vi "GUI.vi"() -> ()   [LabVIEW 2020]
uses:
  <vilib>/Utility/miscctls.llb/LVForegroundBackgroundColorsTypeDef.ctl
  <vilib>/Utility/config.llb/Write Key (String).vi
  <vilib>/Utility/config.llb/Write Key (Boolean).vi
  <vilib>/Utility/config.llb/Write Key (Double).vi
  <vilib>/Utility/config.llb/Write Key (U32).vi
  <vilib>/Utility/config.llb/Read Key (String).vi
  <vilib>/Utility/config.llb/Read Key (Boolean).vi
  <vilib>/Utility/config.llb/Read Key (U32).vi
  <vilib>/Utility/config.llb/Read Key (Double).vi
  <vilib>/Utility/config.llb/NI_LVConfig.lvlib
panel:
  in  "load profiles":bool
  in  "Profile name":string
  in  "Saved profiles":string(combo)
  in  "Save Button":bool
  in  "# channels":dbl=4.0 min=3.0 max=4.0 format="%#_1g"
  in  "To be ignored":dbl=3.0 min=1.0 max=4.0 step=1.0
  in  "RED":dbl=4.0 min=1.0 max=4.0 step=1.0
  in  "GREEN":dbl=1.0 min=1.0 max=4.0 step=1.0
  in  "BLUE":dbl=2.0 min=1.0 max=4.0 step=1.0
  in  "block size":dbl=101.0
  in  "Scroll to last":bool
  in  "Remove Button":bool
  out "Final Scroll Position":i32
  in  "Initial Scroll Position":u32
  out "messages":string
  in  "Red Ch.":bool=TRUE
  in  "Blue Ch.":bool
  in  "Green Ch.":bool=TRUE
  in  "Detailed output":bool
  in  "Python version":string="3.9"
  out "Warning":bool
  out "Error":bool
  out "Warning and error window":string
  out "green static indicator":bool
  out "blue static indicator":bool
  out "red static indicator":bool
  out "Saving":bool
  in  "Overlay Transparency":dbl=0.5 min=0.0 max=1.0 format="%#_3g"
  in  "Activate":bool
  in  "Green":bool
  in  "Blue":bool
  in  "Red":bool
  in  "Green":dbl min=0.0 step=0.001 format="%#_3g"
  in  "Blue":dbl=0.03 min=0.0 step=0.001 format="%#_3g"
  in  "Red":dbl min=0.0 step=0.001 format="%#.3g"
  in  "Green":dbl min=0.0 step=0.001 format="%#_3g"
  in  "Blue":dbl=0.03 min=0.0 step=0.001 format="%#_3g"
  in  "Red":dbl min=0.0 step=0.001 format="%#.3g"
  in  "Green":dbl=1.5 format="%#_2g"
  in  "Blue":dbl=1.5 format="%_2g"
  in  "Red":dbl=1.5 format="%.1g"
  in  "Activate":bool
  in  "Green":dbl=4.0 min=1.0 step=1.0 format="%#_1f"
  in  "Blue":dbl=4.0 min=1.0 step=1.0 format="%_1f"
  in  "Red":dbl=2.0 min=1.0 step=1.0
  in  "Green":bool=TRUE
  in  "Blue":bool=TRUE
  in  "Red":bool=TRUE
  in  "Border thickness (single channel) 2":dbl=1.0 min=1.0 step=1.0 format="%#_3g"
  in  "Activate":bool
  in  "Blue Ch":u32(colorbox)=16711680
  in  "Green Ch":u32(colorbox)=65280
  in  "Red Ch":u32(colorbox)=255
  in  "Red Ch":u32(colorbox)=16776960
  in  "Green Ch":u32(colorbox)=12357519
  in  "Blue Ch":u32(colorbox)=16777215
  in  "Red":dbl=20.0 min=1.0 max=255.0
  in  "Blue":dbl=20.0 min=1.0 max=255.0 format="%_1f"
  in  "Green":dbl=20.0 min=1.0 max=255.0 format="%#_1f"
  in  "Red":dbl=2.0
  in  "Blue":dbl format="%_1f"
  in  "Green":dbl=1.0 format="%#_1f"
  in  "Red":dbl=30000.0 min=2.0 step=1.0
  in  "Blue":dbl=30000.0 min=2.0 step=1.0 format="%_1f"
  in  "Green":dbl=30000.0 min=2.0 step=1.0 format="%#_1f"
  in  "Red":dbl=40.0 min=1.0 step=1.0
  in  "Blue":dbl=40.0 min=1.0 step=1.0 format="%_1f"
  in  "Green":dbl=40.0 min=1.0 step=1.0 format="%#_1f"
  in  "Filling contours by solid color":bool=TRUE
  in  "Border thickness (overlay)":dbl=1.0 format="%#_3g"
  in  "Border thickness (single channel)":dbl=1.0 format="%#_3g"
  in  "General border color":u32(colorbox)=16777215
  in  "Number of bins":dbl=10.0 min=1.0 step=1.0 format="%#_3g"
  out "Processing":bool
  in  "Run":bool
  in  "Green":dbl=2.0 min=1.0 max=3.0 step=1.0 format="%#_1f"
  in  "Blue":dbl=1.0 min=1.0 max=3.0 step=1.0 format="%#_1g"
  in  "Red":dbl=3.0 min=1.0 max=3.0 step=1.0
  in  "Activate Histogram":bool
  in  "Input folder":string="images/"
  in  "Zero Pixel Reporter":bool
  in  "Contour Detail Reporter":bool
  in  "Transparent Corrector":bool=TRUE
  in  "Save":bool
  # "Path information"
  # "Morphological Filter (ellipse and circular)"
  # "Thresholds"
  # "Color Recipe"
  # "Advance Tools"
  # "Global"
  # "Channel to proccess"
  # "Elliptical Ratio Filter"
  # "Biggest contour generator"
  # "Adaptive"
  # "Circular Ratio Filter"
  # "Up to"
  # "biggest"
  # "Morphological Filter (Ratio)"
  # "Order of plot in histogram"
  # "Visual Effects"
  # "Border colors in full map"
  # "Border colors in transparent map"
  # "Selection Filter"
  # "Block Size"
  # "Size Filter"
  # "Process Order"
  # "Messages:"
  # "Minimum size limit"
  # "Maximum size limit"
  # "Designed by Shahab Bahreini"
  # "Warnings:"
  # "ver. 2.0.0"
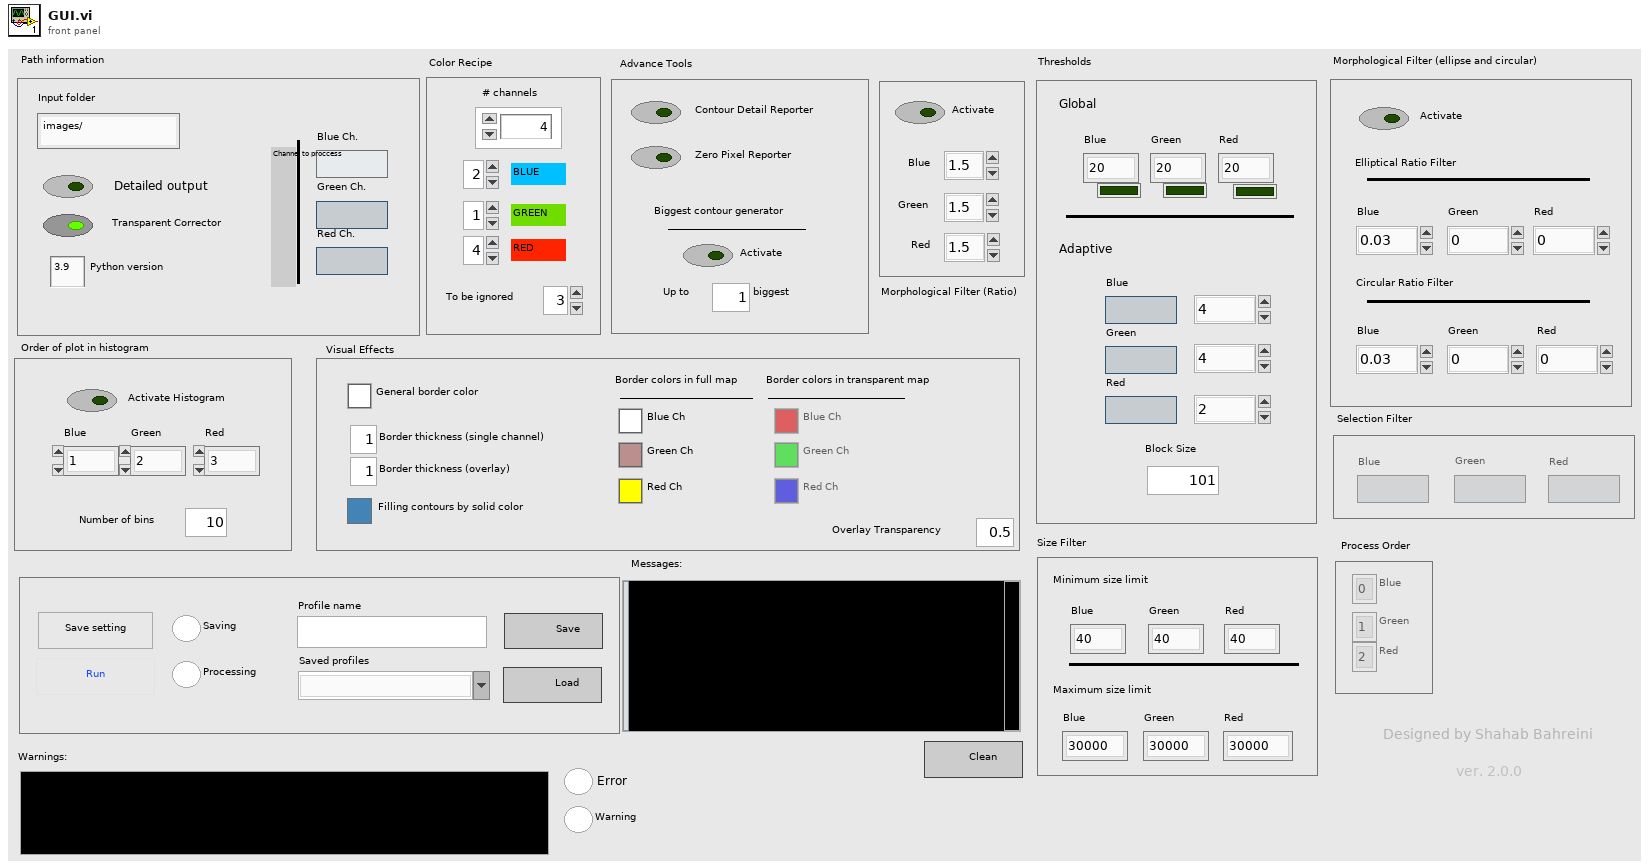
[diagram p1: front panel]
types:
  T1 = enum8{"Enabled", "Disabled", "Disabled and Grayed Out"}
  T2 = typedef "LVForegroundBackgroundColorsTypeDef.ctl" = cluster{"Foreground Color":u32, "Background Color":u32}
  T3 = typedef "NI_LVConfig.lvlib/Config Data RefNum.ctl" = refnum<k1>
  T4 = enum16{"open", "replace", "create", "open or create", "replace or create", "replace or create with confirmation"}
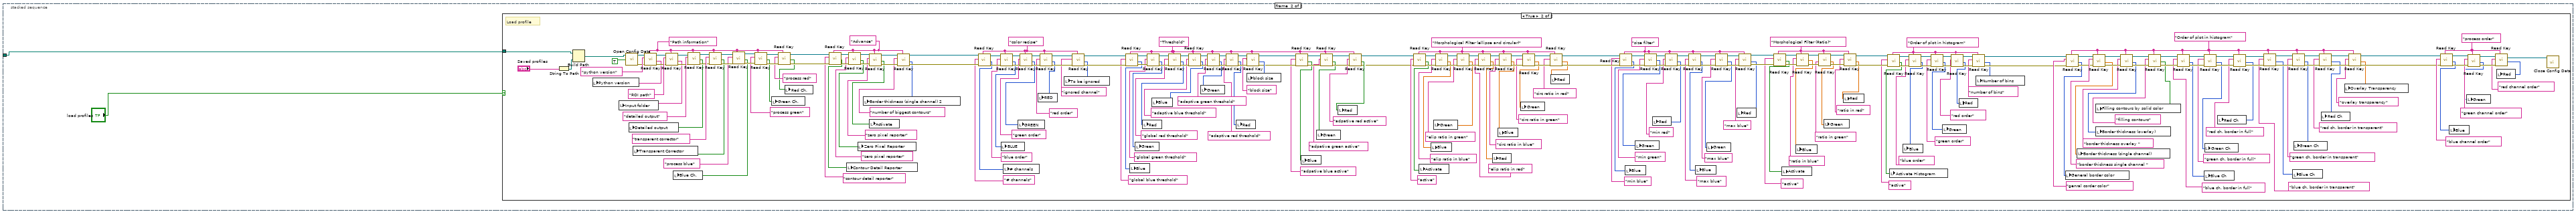
[diagram p3: hidden frame]
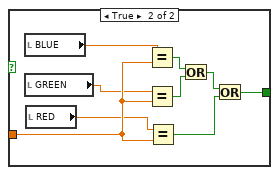
[diagram p5: hidden frame]
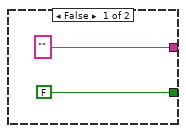
[diagram p6: hidden frame]
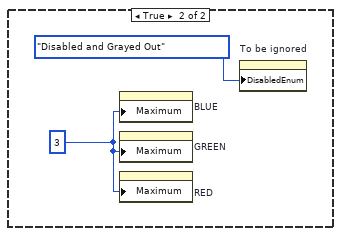
[diagram p7: hidden frame]
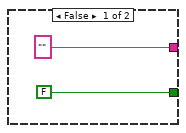
[diagram p9: hidden frame]
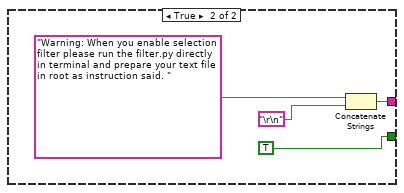
[diagram p10: hidden frame]
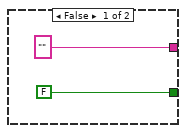
[diagram p11: hidden frame]
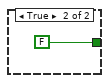
[diagram p12: hidden frame]
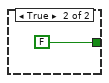
[diagram p13: hidden frame]
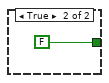
[diagram p14: hidden frame]
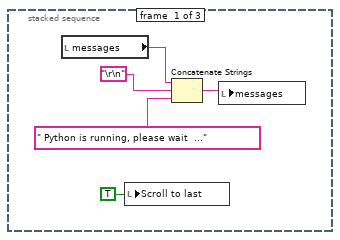
[diagram p16: hidden frame]
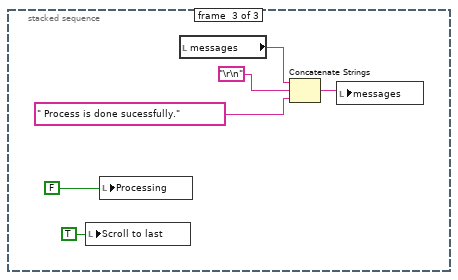
[diagram p17: hidden frame]
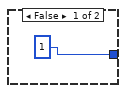
[diagram p19: hidden frame]
diagram:
  # "Finds all .ini profiles"
  # "Recepie error checker"
  # "Selection filter checker"
  # "Size limit checker"
  # "Order of plot checker"
  n1 = local read "Warning and error window"() -> (→"Warning and error window":string)
  n2 = property on="Warning and error window" class="Str"("Text.FontBold"=FALSE ("Text.Font:Bold")) -> ()  [unwired: 2 in, 2 out]
  n3 = property on="Warning and error window" class="Str"("Text.Colors"=T2 {"Foreground Color"=0, "Background Color"=16777222}) -> ()  [unwired: 2 in, 2 out]
  n4 = Equal?(x="# channels", y=3.0) -> (x = y?=w25:bool)
  n5 = case shown="False" w25 {
    frame False {
      w77 = 4
      n6 = property on="BLUE" class="DigNum (strict)"("Maximum"=w77) -> ()  [unwired: 2 in, 2 out]
      n7 = property on="GREEN" class="DigNum (strict)"("Maximum"=w77) -> ()  [unwired: 2 in, 2 out]
      n8 = property on="RED" class="DigNum (strict)"("Maximum"=w77) -> ()  [unwired: 2 in, 2 out]
      n9 = property on="To be ignored" class="DigNum (strict)"("DisabledEnum"=T1."Enabled" ("Disabled")) -> ()  [unwired: 2 in, 2 out]
    }
    frame True {
      w79 = 3
      n10 = property on="BLUE" class="DigNum (strict)"("Maximum"=w79) -> ()  [unwired: 2 in, 2 out]
      n11 = property on="GREEN" class="DigNum (strict)"("Maximum"=w79) -> ()  [unwired: 2 in, 2 out]
      n12 = property on="RED" class="DigNum (strict)"("Maximum"=w79) -> ()  [unwired: 2 in, 2 out]
      n13 = property on="To be ignored" class="DigNum (strict)"("DisabledEnum"=T1."Disabled and Grayed Out" ("Disabled")) -> ()  [unwired: 2 in, 2 out]
    }
  }
  n14 = Current VI's Path() -> (path=w4:path)
  n15 = Strip Path(path=w4) -> (stripped path=w3:path)  [unwired: 1 out]
  n16 = local read "Green"() -> (w71:bool)
  n17 = local read "Blue"() -> (w70:bool)
  n18 = local read "Red"() -> (w72:bool)
  n19 = Build Path(base path=w3, name or relative path=path "profiles") -> (appended path=w1:path)
  n20 = case shown="False" w70 {
    tunnel: [TRUE ("Boolean") FALSE ("Boolean")] -> w68
    frame False {
    }
    frame True {
    }
  }
  "blue static indicator" <- w68
  n21 = case shown="False" w72 {
    tunnel: [TRUE ("Boolean") FALSE ("Boolean")] -> w73
    frame False {
    }
    frame True {
    }
  }
  "red static indicator" <- w73
  n22 = List Folder(path=w1) -> (filenames=w5:string[])  [unwired: 3 in, 3 out]
  n23 = case shown="False" w71 {
    tunnel: [TRUE ("Boolean") FALSE ("Boolean")] -> w69
    frame False {
    }
    frame True {
    }
  }
  "green static indicator" <- w69
  n24 = property on="Saved profiles" class="CmbBox"("Strings[]"=w5) -> ()  [unwired: 2 in, 2 out]
  n25 = local read "To be ignored"() -> (w11:dbl)
  n26 = property on="To be ignored" class="DigNum (strict)"() -> ("DisabledEnum"=w14:T1)  [unwired: 2 in, 2 out]
  n27 = stacked-sequence {
    tunnel: w1 -> [w87 w353]
    frame #0 {
      n28 = case shown="True" "Save Button" {
        tunnel: w87 -> [_ w335]
        frame False {
        }
        frame True {
          w113 = "process order" ("section")
          w142 = "Order of plot in histogram" ("section")
          w183 = "Order of plot in histogram" ("section")
          w184 = "Morphological Filter (Ratio)" ("section")
          w215 = "size filter" ("section")
          w252 = "Morphological Filter (ellipse and circular)" ("section")
          w93 = "Threshold" ("section")
          w279 = "color recipe" ("section")
          w300 = "Advance" ("section")
          w318 = "Path information" ("section")
          # "Save profile"
          n29 = Concatenate Strings("Profile name", ".ini" ("string")) -> (w338:string)
          n30 = String To Path(string=w338) -> (path=w337:path)
          n31 = Build Path(base path=w335, name or relative path=w337) -> (appended path=w340:path)
          n32 = local read "Python version"() -> (w317:string)
          n33 = local read "Input folder"() -> (w345:string)
          n34 = call <vilib>:"Open Config Data.vi"("create file if necessary (T)"=TRUE, "configuration file path"=w340) -> ("error out"=w332:errorcluster, "refnum"=w349:T3)  [unwired: 7 in, 1 out]
          n35 = local read "Detailed output"() -> (w344:bool)
          n36 = local read "Transparent Corrector"() -> (w341:bool)
          n37 = call-poly <vilib>:"Write Key.vi"("section"=w318, "error in (no error)"=w332, "value"=w317, "key"="python version", "refnum"=w349) -> ("error out"=w331:errorcluster, "refnum out"=w352:T3)  [unwired: 4 in, 1 out]
          n38 = local read "Blue Ch."() -> (w327:bool)
          n39 = call-poly <vilib>:"Write Key.vi"("section"=w318, "error in (no error)"=w331, "value"=w345, "key"="ROI path", "refnum"=w352) -> ("error out"=w330:errorcluster, "refnum out"=w351:T3)  [unwired: 4 in, 1 out]
          n40 = call-poly <vilib>:"Write Key.vi"("section"=w318, "error in (no error)"=w330, "value"=w344, "key"="detailed output", "refnum"=w351) -> ("error out"=w329:errorcluster, "refnum out"=w350:T3)  [unwired: 4 in, 1 out]
          n41 = call-poly <vilib>:"Write Key.vi"("section"=w318, "error in (no error)"=w329, "value"=w341, "key"="transparent corrector", "refnum"=w350) -> ("error out"=w334:errorcluster, "refnum out"=w333:T3)  [unwired: 4 in, 1 out]
          n42 = call-poly <vilib>:"Write Key.vi"("section"=w318, "error in (no error)"=w334, "value"=w327, "key"="process blue", "refnum"=w333) -> ("error out"=w324:errorcluster, "refnum out"=w326:T3)  [unwired: 4 in, 1 out]
          n43 = local read "Green Ch."() -> (w319:bool)
          n44 = call-poly <vilib>:"Write Key.vi"("section"=w318, "error in (no error)"=w324, "value"=w319, "key"="process green", "refnum"=w326) -> ("error out"=w323:errorcluster, "refnum out"=w325:T3)  [unwired: 4 in, 1 out]
          n45 = local read "Red Ch."() -> (w321:bool)
          n46 = call-poly <vilib>:"Write Key.vi"("section"=w318, "error in (no error)"=w323, "value"=w321, "key"="process red", "refnum"=w325) -> ("error out"=w315:errorcluster, "refnum out"=w316:T3)  [unwired: 4 in, 1 out]
          n47 = local read "Contour Detail Reporter"() -> (w314:bool)
          n48 = call-poly <vilib>:"Write Key.vi"("section"=w300, "error in (no error)"=w315, "value"=w314, "key"="contour detail reporter", "refnum"=w316) -> ("error out"=w312:errorcluster, "refnum out"=w311:T3)  [unwired: 4 in, 1 out]
          n49 = local read "Zero Pixel Reporter"() -> (w309:bool)
          n50 = call-poly <vilib>:"Write Key.vi"("section"=w300, "error in (no error)"=w312, "value"=w309, "key"="zero pixel reporter", "refnum"=w311) -> ("error out"=w308:errorcluster, "refnum out"=w307:T3)  [unwired: 4 in, 1 out]
          n51 = local read "Activate"() -> (w306:bool)
          n52 = local read "Border thickness (single channel) 2"() -> (w302:dbl)
          n53 = call-poly <vilib>:"Write Key.vi"("section"=w300, "error in (no error)"=w308, "value"=w306, "key"="zero pixel reporter", "refnum"=w307) -> ("error out"=w304:errorcluster, "refnum out"=w303:T3)  [unwired: 4 in, 1 out]
          n54 = call-poly <vilib>:"Write Key.vi"("section"=w300, "error in (no error)"=w304, "value"=w302, "key"="number of biggest contours", "refnum"=w303) -> ("error out"=w295:errorcluster, "refnum out"=w296:T3)  [unwired: 4 in, 1 out]
          n55 = local read "BLUE"() -> (w289:dbl)
          n56 = local read "# channels"() -> (w291:dbl)
          n57 = call-poly <vilib>:"Write Key.vi"("section"=w279, "error in (no error)"=w295, "value"=w291, "key"="# channels", "refnum"=w296) -> ("error out"=w294:errorcluster, "refnum out"=w299:T3)  [unwired: 4 in, 1 out]
          n58 = call-poly <vilib>:"Write Key.vi"("section"=w279, "error in (no error)"=w294, "value"=w289, "key"="blue order", "refnum"=w299) -> ("error out"=w293:errorcluster, "refnum out"=w298:T3)  [unwired: 4 in, 1 out]
          n59 = local read "GREEN"() -> (w286:dbl)
          n60 = call-poly <vilib>:"Write Key.vi"("section"=w279, "error in (no error)"=w293, "value"=w286, "key"="green order", "refnum"=w298) -> ("error out"=w292:errorcluster, "refnum out"=w297:T3)  [unwired: 4 in, 1 out]
          n61 = local read "RED"() -> (w285:dbl)
          n62 = call-poly <vilib>:"Write Key.vi"("section"=w279, "error in (no error)"=w292, "value"=w285, "key"="red order", "refnum"=w297) -> ("error out"=w283:errorcluster, "refnum out"=w282:T3)  [unwired: 4 in, 1 out]
          n63 = local read "To be ignored"() -> (w281:dbl)
          n64 = call-poly <vilib>:"Write Key.vi"("section"=w279, "error in (no error)"=w283, "value"=w281, "key"="ignored channel", "refnum"=w282) -> ("error out"=w267:errorcluster, "refnum out"=w268:T3)  [unwired: 4 in, 1 out]
          n65 = local read "Blue"() -> (w265:dbl)
          n66 = call-poly <vilib>:"Write Key.vi"("section"=w93, "error in (no error)"=w267, "value"=w265, "key"="global blue threshold", "refnum"=w268) -> ("error out"=w273:errorcluster, "refnum out"=w275:T3)  [unwired: 4 in, 1 out]
          n67 = local read "Green"() -> (w263:dbl)
          n68 = local read "Red"() -> (w261:dbl)
          n69 = local read "Blue"() -> (w260:dbl)
          n70 = call-poly <vilib>:"Write Key.vi"("section"=w93, "error in (no error)"=w273, "value"=w263, "key"="global green threshold", "refnum"=w275) -> ("error out"=w272:errorcluster, "refnum out"=w276:T3)  [unwired: 4 in, 1 out]
          n71 = call-poly <vilib>:"Write Key.vi"("section"=w93, "error in (no error)"=w272, "value"=w261, "key"="global red threshold", "refnum"=w276) -> ("error out"=w271:errorcluster, "refnum out"=w277:T3)  [unwired: 4 in, 1 out]
          n72 = call-poly <vilib>:"Write Key.vi"("section"=w93, "error in (no error)"=w271, "value"=w260, "key"="adaptive blue threshold", "refnum"=w277) -> ("error out"=w270:errorcluster, "refnum out"=w278:T3)  [unwired: 4 in, 1 out]
          n73 = local read "Red"() -> (w256:dbl)
          n74 = local read "block size"() -> (w254:dbl)
          n75 = local read "Green"() -> (w258:dbl)
          n76 = call-poly <vilib>:"Write Key.vi"("section"=w93, "error in (no error)"=w270, "value"=w258, "key"="adaptive green threshold", "refnum"=w278) -> ("error out"=w92:errorcluster, "refnum out"=w96:T3)  [unwired: 4 in, 1 out]
          n77 = call-poly <vilib>:"Write Key.vi"("section"=w93, "error in (no error)"=w92, "value"=w256, "key"="adaptive red threshold", "refnum"=w96) -> ("error out"=w269:errorcluster, "refnum out"=w274:T3)  [unwired: 4 in, 1 out]
          n78 = call-poly <vilib>:"Write Key.vi"("section"=w93, "error in (no error)"=w269, "value"=w254, "key"="block size", "refnum"=w274) -> ()  [unwired: 4 in, 3 out]
          n79 = local read "Blue"() -> (w91:bool)
          n80 = call-poly <vilib>:"Write Key.vi"("section"=w93, "error in (no error)"=w92, "value"=w91, "key"="adpative blue active", "refnum"=w96) -> ("error out"=w101:errorcluster, "refnum out"=w103:T3)  [unwired: 4 in, 1 out]
          n81 = local read "Green"() -> (w90:bool)
          n82 = call-poly <vilib>:"Write Key.vi"("section"=w93, "error in (no error)"=w101, "value"=w90, "key"="adpative green active", "refnum"=w103) -> ("error out"=w100:errorcluster, "refnum out"=w102:T3)  [unwired: 4 in, 1 out]
          n83 = local read "Red"() -> (w89:bool)
          n84 = call-poly <vilib>:"Write Key.vi"("section"=w93, "error in (no error)"=w100, "value"=w89, "key"="adpative red active", "refnum"=w102) -> ("error out"=w94:errorcluster, "refnum out"=w95:T3)  [unwired: 4 in, 1 out]
          n85 = local read "Activate"() -> (w238:bool)
          n86 = call-poly <vilib>:"Write Key.vi"("section"=w252, "error in (no error)"=w94, "value"=w238, "key"="active", "refnum"=w95) -> ("error out"=w246:errorcluster, "refnum out"=w243:T3)  [unwired: 4 in, 1 out]
          n87 = local read "Blue"() -> (w236:dbl)
          n88 = local read "Green"() -> (w235:dbl)
          n89 = call-poly <vilib>:"Write Key.vi"("section"=w252, "error in (no error)"=w246, "value"=w236, "key"="elip ratio in blue", "refnum"=w243) -> ("error out"=w247:errorcluster, "refnum out"=w242:T3)  [unwired: 4 in, 1 out]
          n90 = call-poly <vilib>:"Write Key.vi"("section"=w252, "error in (no error)"=w247, "value"=w235, "key"="elip ratio in green", "refnum"=w242) -> ("error out"=w248:errorcluster, "refnum out"=w241:T3)  [unwired: 4 in, 1 out]
          n91 = local read "Red"() -> (w233:dbl)
          n92 = call-poly <vilib>:"Write Key.vi"("section"=w252, "error in (no error)"=w248, "value"=w233, "key"="elip ratio in red", "refnum"=w241) -> ("error out"=w249:errorcluster, "refnum out"=w240:T3)  [unwired: 4 in, 1 out]
          n93 = local read "Blue"() -> (w230:dbl)
          n94 = call-poly <vilib>:"Write Key.vi"("section"=w252, "error in (no error)"=w249, "value"=w230, "key"="circ ratio in blue", "refnum"=w240) -> ("error out"=w250:errorcluster, "refnum out"=w245:T3)  [unwired: 4 in, 1 out]
          n95 = local read "Green"() -> (w229:dbl)
          n96 = call-poly <vilib>:"Write Key.vi"("section"=w252, "error in (no error)"=w250, "value"=w229, "key"="circ ratio in green", "refnum"=w245) -> ("error out"=w251:errorcluster, "refnum out"=w244:T3)  [unwired: 4 in, 1 out]
          n97 = local read "Red"() -> (w226:dbl)
          n98 = call-poly <vilib>:"Write Key.vi"("section"=w252, "error in (no error)"=w251, "value"=w226, "key"="circ ratio in red", "refnum"=w244) -> ("error out"=w213:errorcluster, "refnum out"=w214:T3)  [unwired: 4 in, 1 out]
          n99 = local read "Blue"() -> (w211:dbl)
          n100 = call-poly <vilib>:"Write Key.vi"("section"=w215, "error in (no error)"=w213, "value"=w211, "key"="min blue", "refnum"=w214) -> ("error out"=w220:errorcluster, "refnum out"=w223:T3)  [unwired: 4 in, 1 out]
          n101 = local read "Green"() -> (w209:dbl)
          n102 = call-poly <vilib>:"Write Key.vi"("section"=w215, "error in (no error)"=w220, "value"=w209, "key"="min green", "refnum"=w223) -> ("error out"=w219:errorcluster, "refnum out"=w224:T3)  [unwired: 4 in, 1 out]
          n103 = local read "Red"() -> (w208:dbl)
          n104 = call-poly <vilib>:"Write Key.vi"("section"=w215, "error in (no error)"=w219, "value"=w208, "key"="min red", "refnum"=w224) -> ("error out"=w218:errorcluster, "refnum out"=w225:T3)  [unwired: 4 in, 1 out]
          n105 = local read "Blue"() -> (w205:dbl)
          n106 = call-poly <vilib>:"Write Key.vi"("section"=w215, "error in (no error)"=w218, "value"=w205, "key"="max blue", "refnum"=w225) -> ("error out"=w217:errorcluster, "refnum out"=w221:T3)  [unwired: 4 in, 1 out]
          n107 = local read "Green"() -> (w203:dbl)
          n108 = call-poly <vilib>:"Write Key.vi"("section"=w215, "error in (no error)"=w217, "value"=w203, "key"="max blue", "refnum"=w221) -> ("error out"=w216:errorcluster, "refnum out"=w222:T3)  [unwired: 4 in, 1 out]
          n109 = local read "Red"() -> (w201:dbl)
          n110 = call-poly <vilib>:"Write Key.vi"("section"=w215, "error in (no error)"=w216, "value"=w201, "key"="max blue", "refnum"=w222) -> ("error out"=w195:errorcluster, "refnum out"=w196:T3)  [unwired: 4 in, 1 out]
          n111 = local read "Activate"() -> (w191:bool)
          n112 = call-poly <vilib>:"Write Key.vi"("section"=w184, "error in (no error)"=w195, "value"=w191, "key"="active", "refnum"=w196) -> ("error out"=w199:errorcluster, "refnum out"=w198:T3)  [unwired: 4 in, 1 out]
          n113 = local read "Blue"() -> (w189:dbl)
          n114 = call-poly <vilib>:"Write Key.vi"("section"=w184, "error in (no error)"=w199, "value"=w189, "key"="ratio in blue", "refnum"=w198) -> ("error out"=w200:errorcluster, "refnum out"=w197:T3)  [unwired: 4 in, 1 out]
          n115 = local read "Green"() -> (w187:dbl)
          n116 = call-poly <vilib>:"Write Key.vi"("section"=w184, "error in (no error)"=w200, "value"=w187, "key"="ratio in green", "refnum"=w197) -> ("error out"=w193:errorcluster, "refnum out"=w194:T3)  [unwired: 4 in, 1 out]
          n117 = local read "Red"() -> (w186:dbl)
          n118 = call-poly <vilib>:"Write Key.vi"("section"=w184, "error in (no error)"=w193, "value"=w186, "key"="ratio in red", "refnum"=w194) -> ("error out"=w173:errorcluster, "refnum out"=w174:T3)  [unwired: 4 in, 1 out]
          n119 = local read "Activate Histogram"() -> (w172:bool)
          n120 = call-poly <vilib>:"Write Key.vi"("section"=w183, "error in (no error)"=w173, "value"=w172, "key"="active", "refnum"=w174) -> ("error out"=w179:errorcluster, "refnum out"=w177:T3)  [unwired: 4 in, 1 out]
          n121 = local read "Blue"() -> (w169:dbl)
          n122 = call-poly <vilib>:"Write Key.vi"("section"=w183, "error in (no error)"=w179, "value"=w169, "key"="blue order", "refnum"=w177) -> ("error out"=w180:errorcluster, "refnum out"=w176:T3)  [unwired: 4 in, 1 out]
          n123 = local read "Green"() -> (w167:dbl)
          n124 = call-poly <vilib>:"Write Key.vi"("section"=w183, "error in (no error)"=w180, "value"=w167, "key"="green order", "refnum"=w176) -> ("error out"=w181:errorcluster, "refnum out"=w175:T3)  [unwired: 4 in, 1 out]
          n125 = local read "Red"() -> (w165:dbl)
          n126 = call-poly <vilib>:"Write Key.vi"("section"=w183, "error in (no error)"=w181, "value"=w165, "key"="red order", "refnum"=w175) -> ("error out"=w182:errorcluster, "refnum out"=w178:T3)  [unwired: 4 in, 1 out]
          n127 = local read "Number of bins"() -> (w163:dbl)
          n128 = call-poly <vilib>:"Write Key.vi"("section"=w183, "error in (no error)"=w182, "value"=w163, "key"="number of bins", "refnum"=w178) -> ("error out"=w118:errorcluster, "refnum out"=w119:T3)  [unwired: 4 in, 1 out]
          n129 = local read "General border color"() -> (w140:u32)
          n130 = call-poly <vilib>:"Write Key.vi"("section"=w142, "error in (no error)"=w118, "value"=w140, "key"="genral corder color", "refnum"=w119) -> ("error out"=w158:errorcluster, "refnum out"=w160:T3)  [unwired: 4 in, 1 out]
          n131 = local read "Border thickness (single channel)"() -> (w138:dbl)
          n132 = local read "Filling contours by solid color"() -> (w135:bool)
          n133 = call-poly <vilib>:"Write Key.vi"("section"=w142, "error in (no error)"=w158, "value"=w138, "key"="border thickness single channel ", "refnum"=w160) -> ("error out"=w157:errorcluster, "refnum out"=w161:T3)  [unwired: 4 in, 1 out]
          n134 = local read "Border thickness (overlay)"() -> (w137:dbl)
          n135 = call-poly <vilib>:"Write Key.vi"("section"=w142, "error in (no error)"=w157, "value"=w137, "key"="border thickness overlay ", "refnum"=w161) -> ("error out"=w156:errorcluster, "refnum out"=w162:T3)  [unwired: 4 in, 1 out]
          n136 = call-poly <vilib>:"Write Key.vi"("section"=w142, "error in (no error)"=w156, "value"=w135, "key"="filling contours", "refnum"=w162) -> ("error out"=w155:errorcluster, "refnum out"=w159:T3)  [unwired: 4 in, 1 out]
          n137 = local read "Blue Ch"() -> (w132:u32)
          n138 = call-poly <vilib>:"Write Key.vi"("section"=w142, "error in (no error)"=w155, "value"=w132, "key"="blue ch. border in full", "refnum"=w159) -> ("error out"=w154:errorcluster, "refnum out"=w153:T3)  [unwired: 4 in, 1 out]
          n139 = local read "Green Ch"() -> (w130:u32)
          n140 = call-poly <vilib>:"Write Key.vi"("section"=w142, "error in (no error)"=w154, "value"=w130, "key"="green ch. border in full", "refnum"=w153) -> ("error out"=w152:errorcluster, "refnum out"=w151:T3)  [unwired: 4 in, 1 out]
          n141 = local read "Red Ch"() -> (w128:u32)
          n142 = call-poly <vilib>:"Write Key.vi"("section"=w142, "error in (no error)"=w152, "value"=w128, "key"="red ch. border in full", "refnum"=w151) -> ("error out"=w144:errorcluster, "refnum out"=w143:T3)  [unwired: 4 in, 1 out]
          n143 = local read "Blue Ch"() -> (w126:u32)
          n144 = call-poly <vilib>:"Write Key.vi"("section"=w142, "error in (no error)"=w144, "value"=w126, "key"="blue ch. border in transparent", "refnum"=w143) -> ("error out"=w146:errorcluster, "refnum out"=w145:T3)  [unwired: 4 in, 1 out]
          n145 = local read "Green Ch"() -> (w124:u32)
          n146 = call-poly <vilib>:"Write Key.vi"("section"=w142, "error in (no error)"=w146, "value"=w124, "key"="green ch. border in transparent", "refnum"=w145) -> ("error out"=w147:errorcluster, "refnum out"=w148:T3)  [unwired: 4 in, 1 out]
          n147 = local read "Red Ch"() -> (w122:u32)
          n148 = call-poly <vilib>:"Write Key.vi"("section"=w142, "error in (no error)"=w147, "value"=w122, "key"="red ch. border in transparent", "refnum"=w148) -> ("error out"=w149:errorcluster, "refnum out"=w150:T3)  [unwired: 4 in, 1 out]
          n149 = local read "Overlay Transparency"() -> (w120:dbl)
          n150 = call-poly <vilib>:"Write Key.vi"("section"=w142, "error in (no error)"=w149, "value"=w120, "key"="overlay transparency", "refnum"=w150) -> ("error out"=w105:errorcluster, "refnum out"=w106:T3)  [unwired: 4 in, 1 out]
          n151 = local read "Blue"() -> (w110:dbl)
          n152 = call-poly <vilib>:"Write Key.vi"("section"=w113, "error in (no error)"=w105, "value"=w110, "key"="blue channel order", "refnum"=w106) -> ("error out"=w116:errorcluster, "refnum out"=w117:T3)  [unwired: 4 in, 1 out]
          n153 = local read "Green"() -> (w112:dbl)
          n154 = call-poly <vilib>:"Write Key.vi"("section"=w113, "error in (no error)"=w116, "value"=w112, "key"="green channel order", "refnum"=w117) -> ("error out"=w115:errorcluster, "refnum out"=w114:T3)  [unwired: 4 in, 1 out]
          n155 = local read "Red"() -> (w111:dbl)
          n156 = call-poly <vilib>:"Write Key.vi"("section"=w113, "error in (no error)"=w115, "value"=w111, "key"="red channel order", "refnum"=w114) -> ("refnum out"=w104:T3)  [unwired: 4 in, 2 out]
          n157 = call <vilib>:"Close Config Data.vi"("refnum"=w104) -> ()  [unwired: 9 in, 2 out]
        }
      }
    }
    frame #1 {
      n158 = case shown="True" "load profiles" {
        tunnel: w353 -> [_ w607]
        frame False {
        }
        frame True {
          w438 = "process order" ("section")
          w455 = "Order of plot in histogram" ("section")
          w490 = "Order of plot in histogram" ("section")
          w491 = "Morphological Filter (Ratio)" ("section")
          w512 = "size filter" ("section")
          w542 = "Morphological Filter (ellipse and circular)" ("section")
          w363 = "Threshold" ("section")
          w564 = "color recipe" ("section")
          w580 = "Advance" ("section")
          w593 = "Path information" ("section")
          # "Load profile"
          n159 = String To Path(string="Saved profiles") -> (path=w608:path)
          n160 = Build Path(base path=w607, name or relative path=w608) -> (appended path=w609:path)
          n161 = call <vilib>:"Open Config Data.vi"("create file if necessary (T)"=TRUE, "configuration file path"=w609) -> ("error out"=w604:errorcluster, "refnum"=w615:T3)  [unwired: 7 in, 1 out]
          n162 = call-poly <vilib>:"Read Key.vi"("section"=w593, "error in (no error)"=w604, "key"="python version", "refnum"=w615) -> ("error out"=w603:errorcluster, "value"=w431:string, "refnum out"=w618:T3)  [unwired: 4 in, 1 out]
          n163 = local write "Python version"(w431) -> ()
          n164 = call-poly <vilib>:"Read Key.vi"("section"=w593, "error in (no error)"=w603, "key"="ROI path", "refnum"=w618) -> ("error out"=w602:errorcluster, "value"=w430:string, "refnum out"=w617:T3)  [unwired: 4 in, 1 out]
          n165 = local write "Input folder"(w430) -> ()
          n166 = call-poly <vilib>:"Read Key.vi"("section"=w593, "error in (no error)"=w602, "key"="detailed output", "refnum"=w617) -> ("error out"=w601:errorcluster, "value"=w429:bool, "refnum out"=w616:T3)  [unwired: 4 in, 1 out]
          n167 = local write "Detailed output"(w429) -> ()
          n168 = call-poly <vilib>:"Read Key.vi"("section"=w593, "error in (no error)"=w601, "key"="transparent corrector", "refnum"=w616) -> ("error out"=w606:errorcluster, "value"=w428:bool, "refnum out"=w605:T3)  [unwired: 4 in, 1 out]
          n169 = local write "Transparent Corrector"(w428) -> ()
          n170 = call-poly <vilib>:"Read Key.vi"("section"=w593, "error in (no error)"=w606, "key"="process blue", "refnum"=w605) -> ("error out"=w597:errorcluster, "value"=w427:bool, "refnum out"=w599:T3)  [unwired: 4 in, 1 out]
          n171 = local write "Blue Ch."(w427) -> ()
          n172 = call-poly <vilib>:"Read Key.vi"("section"=w593, "error in (no error)"=w597, "key"="process green", "refnum"=w599) -> ("error out"=w596:errorcluster, "value"=w426:bool, "refnum out"=w598:T3)  [unwired: 4 in, 1 out]
          n173 = local write "Green Ch."(w426) -> ()
          n174 = call-poly <vilib>:"Read Key.vi"("section"=w593, "error in (no error)"=w596, "key"="process red", "refnum"=w598) -> ("error out"=w591:errorcluster, "value"=w425:bool, "refnum out"=w592:T3)  [unwired: 4 in, 1 out]
          n175 = local write "Red Ch."(w425) -> ()
          n176 = call-poly <vilib>:"Read Key.vi"("section"=w580, "error in (no error)"=w591, "key"="contour detail reporter", "refnum"=w592) -> ("error out"=w589:errorcluster, "value"=w424:bool, "refnum out"=w588:T3)  [unwired: 4 in, 1 out]
          n177 = local write "Contour Detail Reporter"(w424) -> ()
          n178 = call-poly <vilib>:"Read Key.vi"("section"=w580, "error in (no error)"=w589, "key"="zero pixel reporter", "refnum"=w588) -> ("error out"=w586:errorcluster, "value"=w423:bool, "refnum out"=w585:T3)  [unwired: 4 in, 1 out]
          n179 = local write "Zero Pixel Reporter"(w423) -> ()
          n180 = call-poly <vilib>:"Read Key.vi"("section"=w580, "error in (no error)"=w586, "key"="zero pixel reporter", "refnum"=w585) -> ("error out"=w583:errorcluster, "value"=w422:bool, "refnum out"=w582:T3)  [unwired: 4 in, 1 out]
          n181 = local write "Activate"(w422) -> ()
          n182 = call-poly <vilib>:"Read Key.vi"("section"=w580, "error in (no error)"=w583, "key"="number of biggest contours", "refnum"=w582) -> ("error out"=w575:errorcluster, "value"=w421:u32, "refnum out"=w576:T3)  [unwired: 4 in, 1 out]
          n183 = local write "Border thickness (single channel) 2"(w421) -> ()
          n184 = call-poly <vilib>:"Read Key.vi"("section"=w564, "error in (no error)"=w575, "key"="# channels", "refnum"=w576) -> ("error out"=w574:errorcluster, "value"=w420:u32, "refnum out"=w579:T3)  [unwired: 4 in, 1 out]
          n185 = call-poly <vilib>:"Read Key.vi"("section"=w564, "error in (no error)"=w574, "key"="blue order", "refnum"=w579) -> ("error out"=w573:errorcluster, "value"=w419:u32, "refnum out"=w578:T3)  [unwired: 4 in, 1 out]
          n186 = local write "BLUE"(w419) -> ()
          n187 = local write "# channels"(w420) -> ()
          n188 = call-poly <vilib>:"Read Key.vi"("section"=w564, "error in (no error)"=w573, "key"="green order", "refnum"=w578) -> ("error out"=w572:errorcluster, "value"=w418:u32, "refnum out"=w577:T3)  [unwired: 4 in, 1 out]
          n189 = local write "GREEN"(w418) -> ()
          n190 = call-poly <vilib>:"Read Key.vi"("section"=w564, "error in (no error)"=w572, "key"="red order", "refnum"=w577) -> ("error out"=w567:errorcluster, "value"=w417:u32, "refnum out"=w566:T3)  [unwired: 4 in, 1 out]
          n191 = local write "RED"(w417) -> ()
          n192 = call-poly <vilib>:"Read Key.vi"("section"=w564, "error in (no error)"=w567, "key"="ignored channel", "refnum"=w566) -> ("error out"=w550:errorcluster, "value"=w416:u32, "refnum out"=w551:T3)  [unwired: 4 in, 1 out]
          n193 = local write "To be ignored"(w416) -> ()
          n194 = call-poly <vilib>:"Read Key.vi"("section"=w363, "error in (no error)"=w550, "key"="global blue threshold", "refnum"=w551) -> ("error out"=w557:errorcluster, "value"=w415:u32, "refnum out"=w560:T3)  [unwired: 4 in, 1 out]
          n195 = local write "Blue"(w415) -> ()
          n196 = call-poly <vilib>:"Read Key.vi"("section"=w363, "error in (no error)"=w557, "key"="global green threshold", "refnum"=w560) -> ("error out"=w556:errorcluster, "value"=w414:u32, "refnum out"=w561:T3)  [unwired: 4 in, 1 out]
          n197 = local write "Green"(w414) -> ()
          n198 = call-poly <vilib>:"Read Key.vi"("section"=w363, "error in (no error)"=w556, "key"="global red threshold", "refnum"=w561) -> ("error out"=w555:errorcluster, "value"=w413:u32, "refnum out"=w562:T3)  [unwired: 4 in, 1 out]
          n199 = local write "Red"(w413) -> ()
          n200 = call-poly <vilib>:"Read Key.vi"("section"=w363, "error in (no error)"=w555, "key"="adaptive blue threshold", "refnum"=w562) -> ("error out"=w554:errorcluster, "value"=w412:u32, "refnum out"=w563:T3)  [unwired: 4 in, 1 out]
          n201 = local write "Blue"(w412) -> ()
          n202 = call-poly <vilib>:"Read Key.vi"("section"=w363, "error in (no error)"=w554, "key"="adaptive green threshold", "refnum"=w563) -> ("error out"=w553:errorcluster, "value"=w411:u32, "refnum out"=w558:T3)  [unwired: 4 in, 1 out]
          n203 = local write "Green"(w411) -> ()
          n204 = call-poly <vilib>:"Read Key.vi"("section"=w363, "error in (no error)"=w553, "key"="adaptive red threshold", "refnum"=w558) -> ("error out"=w552:errorcluster, "value"=w410:u32, "refnum out"=w559:T3)  [unwired: 4 in, 1 out]
          n205 = local write "Red"(w410) -> ()
          n206 = call-poly <vilib>:"Read Key.vi"("section"=w363, "error in (no error)"=w552, "key"="block size", "refnum"=w559) -> ("error out"=w367:errorcluster, "value"=w409:u32, "refnum out"=w364:T3)  [unwired: 4 in, 1 out]
          n207 = local write "block size"(w409) -> ()
          n208 = call-poly <vilib>:"Read Key.vi"("section"=w363, "error in (no error)"=w367, "key"="adpative blue active", "refnum"=w364) -> ("error out"=w366:errorcluster, "value"=w361:bool, "refnum out"=w369:T3)  [unwired: 4 in, 1 out]
          n209 = local write "Blue"(w361) -> ()
          n210 = call-poly <vilib>:"Read Key.vi"("section"=w363, "error in (no error)"=w366, "key"="adpative green active", "refnum"=w369) -> ("error out"=w365:errorcluster, "value"=w360:bool, "refnum out"=w368:T3)  [unwired: 4 in, 1 out]
          n211 = local write "Green"(w360) -> ()
          n212 = call-poly <vilib>:"Read Key.vi"("section"=w363, "error in (no error)"=w365, "key"="adpative red active", "refnum"=w368) -> ("error out"=w356:errorcluster, "value"=w358:bool, "refnum out"=w355:T3)  [unwired: 4 in, 1 out]
          n213 = local write "Red"(w358) -> ()
          n214 = call-poly <vilib>:"Read Key.vi"("section"=w542, "error in (no error)"=w356, "key"="active", "refnum"=w355) -> ("error out"=w536:errorcluster, "value"=w408:bool, "refnum out"=w533:T3)  [unwired: 4 in, 1 out]
          n215 = local write "Activate"(w408) -> ()
          n216 = call-poly <vilib>:"Read Key.vi"("section"=w542, "error in (no error)"=w536, "key"="elip ratio in blue", "refnum"=w533) -> ("error out"=w537:errorcluster, "value"=w407:dbl, "refnum out"=w532:T3)  [unwired: 4 in, 1 out]
          n217 = local write "Blue"(w407) -> ()
          n218 = call-poly <vilib>:"Read Key.vi"("section"=w542, "error in (no error)"=w537, "key"="elip ratio in green", "refnum"=w532) -> ("error out"=w538:errorcluster, "value"=w406:dbl, "refnum out"=w531:T3)  [unwired: 4 in, 1 out]
          n219 = local write "Green"(w406) -> ()
          n220 = call-poly <vilib>:"Read Key.vi"("section"=w542, "error in (no error)"=w538, "key"="elip ratio in red", "refnum"=w531) -> ("error out"=w539:errorcluster, "value"=w405:dbl, "refnum out"=w530:T3)  [unwired: 4 in, 1 out]
          n221 = local write "Red"(w405) -> ()
          n222 = call-poly <vilib>:"Read Key.vi"("section"=w542, "error in (no error)"=w539, "key"="circ ratio in blue", "refnum"=w530) -> ("error out"=w540:errorcluster, "value"=w404:dbl, "refnum out"=w535:T3)  [unwired: 4 in, 1 out]
          n223 = local write "Blue"(w404) -> ()
          n224 = call-poly <vilib>:"Read Key.vi"("section"=w542, "error in (no error)"=w540, "key"="circ ratio in green", "refnum"=w535) -> ("error out"=w541:errorcluster, "value"=w403:dbl, "refnum out"=w534:T3)  [unwired: 4 in, 1 out]
          n225 = local write "Green"(w403) -> ()
          n226 = call-poly <vilib>:"Read Key.vi"("section"=w542, "error in (no error)"=w541, "key"="circ ratio in red", "refnum"=w534) -> ("error out"=w510:errorcluster, "value"=w402:dbl, "refnum out"=w511:T3)  [unwired: 4 in, 1 out]
          n227 = local write "Red"(w402) -> ()
          n228 = call-poly <vilib>:"Read Key.vi"("section"=w512, "error in (no error)"=w510, "key"="min blue", "refnum"=w511) -> ("error out"=w517:errorcluster, "value"=w401:u32, "refnum out"=w520:T3)  [unwired: 4 in, 1 out]
          n229 = local write "Blue"(w401) -> ()
          n230 = call-poly <vilib>:"Read Key.vi"("section"=w512, "error in (no error)"=w517, "key"="min green", "refnum"=w520) -> ("error out"=w516:errorcluster, "value"=w400:u32, "refnum out"=w521:T3)  [unwired: 4 in, 1 out]
          n231 = local write "Green"(w400) -> ()
          n232 = call-poly <vilib>:"Read Key.vi"("section"=w512, "error in (no error)"=w516, "key"="min red", "refnum"=w521) -> ("error out"=w515:errorcluster, "value"=w399:u32, "refnum out"=w522:T3)  [unwired: 4 in, 1 out]
          n233 = local write "Red"(w399) -> ()
          n234 = call-poly <vilib>:"Read Key.vi"("section"=w512, "error in (no error)"=w515, "key"="max blue", "refnum"=w522) -> ("error out"=w514:errorcluster, "value"=w398:u32, "refnum out"=w518:T3)  [unwired: 4 in, 1 out]
          n235 = local write "Blue"(w398) -> ()
          n236 = call-poly <vilib>:"Read Key.vi"("section"=w512, "error in (no error)"=w514, "key"="max blue", "refnum"=w518) -> ("error out"=w513:errorcluster, "value"=w397:u32, "refnum out"=w519:T3)  [unwired: 4 in, 1 out]
          n237 = local write "Green"(w397) -> ()
          n238 = call-poly <vilib>:"Read Key.vi"("section"=w512, "error in (no error)"=w513, "key"="max blue", "refnum"=w519) -> ("error out"=w498:errorcluster, "value"=w396:u32, "refnum out"=w499:T3)  [unwired: 4 in, 1 out]
          n239 = local write "Red"(w396) -> ()
          n240 = call-poly <vilib>:"Read Key.vi"("section"=w491, "error in (no error)"=w498, "key"="active", "refnum"=w499) -> ("error out"=w502:errorcluster, "value"=w395:bool, "refnum out"=w501:T3)  [unwired: 4 in, 1 out]
          n241 = local write "Activate"(w395) -> ()
          n242 = call-poly <vilib>:"Read Key.vi"("section"=w491, "error in (no error)"=w502, "key"="ratio in blue", "refnum"=w501) -> ("error out"=w503:errorcluster, "value"=w394:dbl, "refnum out"=w500:T3)  [unwired: 4 in, 1 out]
          n243 = local write "Blue"(w394) -> ()
          n244 = call-poly <vilib>:"Read Key.vi"("section"=w491, "error in (no error)"=w503, "key"="ratio in green", "refnum"=w500) -> ("error out"=w496:errorcluster, "value"=w393:dbl, "refnum out"=w497:T3)  [unwired: 4 in, 1 out]
          n245 = local write "Green"(w393) -> ()
          n246 = call-poly <vilib>:"Read Key.vi"("section"=w491, "error in (no error)"=w496, "key"="ratio in red", "refnum"=w497) -> ("error out"=w480:errorcluster, "value"=w392:dbl, "refnum out"=w481:T3)  [unwired: 4 in, 1 out]
          n247 = local write "Red"(w392) -> ()
          n248 = call-poly <vilib>:"Read Key.vi"("section"=w490, "error in (no error)"=w480, "key"="active", "refnum"=w481) -> ("error out"=w486:errorcluster, "value"=w391:bool, "refnum out"=w484:T3)  [unwired: 4 in, 1 out]
          n249 = local write "Activate Histogram"(w391) -> ()
          n250 = call-poly <vilib>:"Read Key.vi"("section"=w490, "error in (no error)"=w486, "key"="blue order", "refnum"=w484) -> ("error out"=w487:errorcluster, "value"=w390:u32, "refnum out"=w483:T3)  [unwired: 4 in, 1 out]
          n251 = local write "Blue"(w390) -> ()
          n252 = call-poly <vilib>:"Read Key.vi"("section"=w490, "error in (no error)"=w487, "key"="green order", "refnum"=w483) -> ("error out"=w488:errorcluster, "value"=w389:u32, "refnum out"=w482:T3)  [unwired: 4 in, 1 out]
          n253 = local write "Green"(w389) -> ()
          n254 = call-poly <vilib>:"Read Key.vi"("section"=w490, "error in (no error)"=w488, "key"="red order", "refnum"=w482) -> ("error out"=w489:errorcluster, "value"=w388:u32, "refnum out"=w485:T3)  [unwired: 4 in, 1 out]
          n255 = local write "Red"(w388) -> ()
          n256 = call-poly <vilib>:"Read Key.vi"("section"=w490, "error in (no error)"=w489, "key"="number of bins", "refnum"=w485) -> ("error out"=w443:errorcluster, "value"=w387:u32, "refnum out"=w444:T3)  [unwired: 4 in, 1 out]
          n257 = local write "Number of bins"(w387) -> ()
          n258 = call-poly <vilib>:"Read Key.vi"("section"=w455, "error in (no error)"=w443, "key"="genral corder color", "refnum"=w444) -> ("error out"=w372:errorcluster, "value"=w371:u32, "refnum out"=w472:T3)  [unwired: 4 in, 1 out]
          n259 = local write "General border color"(w371) -> ()
          n260 = call-poly <vilib>:"Read Key.vi"("section"=w455, "error in (no error)"=w372, "key"="border thickness single channel ", "refnum"=w472) -> ("error out"=w470:errorcluster, "value"=w373:dbl, "refnum out"=w473:T3)  [unwired: 4 in, 1 out]
          n261 = local write "Border thickness (single channel)"(w373) -> ()
          n262 = call-poly <vilib>:"Read Key.vi"("section"=w455, "error in (no error)"=w470, "key"="border thickness overlay ", "refnum"=w473) -> ("error out"=w469:errorcluster, "value"=w374:u32, "refnum out"=w474:T3)  [unwired: 4 in, 1 out]
          n263 = local write "Border thickness (overlay)"(w374) -> ()
          n264 = call-poly <vilib>:"Read Key.vi"("section"=w455, "error in (no error)"=w469, "key"="filling contours", "refnum"=w474) -> ("error out"=w468:errorcluster, "value"=w376:bool, "refnum out"=w471:T3)  [unwired: 4 in, 1 out]
          n265 = local write "Filling contours by solid color"(w376) -> ()
          n266 = call-poly <vilib>:"Read Key.vi"("section"=w455, "error in (no error)"=w468, "key"="blue ch. border in full", "refnum"=w471) -> ("error out"=w467:errorcluster, "value"=w377:u32, "refnum out"=w466:T3)  [unwired: 4 in, 1 out]
          n267 = call-poly <vilib>:"Read Key.vi"("section"=w455, "error in (no error)"=w467, "key"="green ch. border in full", "refnum"=w466) -> ("error out"=w465:errorcluster, "value"=w378:u32, "refnum out"=w464:T3)  [unwired: 4 in, 1 out]
          n268 = local write "Blue Ch"(w377) -> ()
          n269 = local write "Green Ch"(w378) -> ()
          n270 = call-poly <vilib>:"Read Key.vi"("section"=w455, "error in (no error)"=w465, "key"="red ch. border in full", "refnum"=w464) -> ("error out"=w457:errorcluster, "value"=w379:u32, "refnum out"=w456:T3)  [unwired: 4 in, 1 out]
          n271 = local write "Red Ch"(w379) -> ()
          n272 = call-poly <vilib>:"Read Key.vi"("section"=w455, "error in (no error)"=w457, "key"="blue ch. border in transparent", "refnum"=w456) -> ("error out"=w459:errorcluster, "value"=w380:u32, "refnum out"=w458:T3)  [unwired: 4 in, 1 out]
          n273 = call-poly <vilib>:"Read Key.vi"("section"=w455, "error in (no error)"=w459, "key"="green ch. border in transparent", "refnum"=w458) -> ("error out"=w460:errorcluster, "value"=w381:u32, "refnum out"=w461:T3)  [unwired: 4 in, 1 out]
          n274 = local write "Blue Ch"(w380) -> ()
          n275 = local write "Green Ch"(w381) -> ()
          n276 = call-poly <vilib>:"Read Key.vi"("section"=w455, "error in (no error)"=w460, "key"="red ch. border in transparent", "refnum"=w461) -> ("error out"=w462:errorcluster, "value"=w382:u32, "refnum out"=w463:T3)  [unwired: 4 in, 1 out]
          n277 = local write "Red Ch"(w382) -> ()
          n278 = call-poly <vilib>:"Read Key.vi"("section"=w455, "error in (no error)"=w462, "key"="overlay transparency", "refnum"=w463) -> ("error out"=w433:errorcluster, "value"=w383:dbl, "refnum out"=w434:T3)  [unwired: 4 in, 1 out]
          n279 = local write "Overlay Transparency"(w383) -> ()
          n280 = call-poly <vilib>:"Read Key.vi"("section"=w438, "error in (no error)"=w433, "key"="blue channel order", "refnum"=w434) -> ("error out"=w441:errorcluster, "value"=w386:u32, "refnum out"=w442:T3)  [unwired: 4 in, 1 out]
          n281 = local write "Blue"(w386) -> ()
          n282 = call-poly <vilib>:"Read Key.vi"("section"=w438, "error in (no error)"=w441, "key"="green channel order", "refnum"=w442) -> ("error out"=w440:errorcluster, "value"=w385:u32, "refnum out"=w439:T3)  [unwired: 4 in, 1 out]
          n283 = local write "Green"(w385) -> ()
          n284 = call-poly <vilib>:"Read Key.vi"("section"=w438, "error in (no error)"=w440, "key"="red channel order", "refnum"=w439) -> ("value"=w384:u32, "refnum out"=w432:T3)  [unwired: 4 in, 2 out]
          n285 = local write "Red"(w384) -> ()
          n286 = call <vilib>:"Close Config Data.vi"("refnum"=w432) -> ()  [unwired: 9 in, 2 out]
        }
      }
    }
  }
  n287 = Equal?(x=w14, y=T1."Enabled") -> (x = y?=w12:bool)
  n288 = local read "GREEN"() -> (w16:dbl)
  n289 = local read "BLUE"() -> (w17:dbl)
  n290 = local read "RED"() -> (w15:dbl)
  n291 = case shown="False" w12 {
    tunnel: w11 -> [_ w628]
    tunnel: [FALSE w620] -> w10
    frame False {
    }
    frame True {
      n292 = local read "BLUE"() -> (w627:dbl)
      n293 = local read "GREEN"() -> (w626:dbl)
      n294 = local read "RED"() -> (w625:dbl)
      n295 = Equal?(x=w627, y=w628) -> (x = y?=w624:bool)
      n296 = Equal?(x=w626, y=w628) -> (x = y?=w623:bool)
      n297 = Equal?(x=w625, y=w628) -> (x = y?=w621:bool)
      n298 = Or(x=w624, y=w623) -> (x .or. y?=w622:bool)
      n299 = Or(x=w622, y=w621) -> (x .or. y?=w620:bool)
    }
  }
  n300 = local read "Red"() -> (w67:dbl)
  n301 = local read "Blue"() -> (w66:dbl)
  n302 = local read "Green"() -> (w65:dbl)
  n303 = local read "Red"() -> (w39:dbl)
  n304 = local read "Red"() -> (w47:dbl)
  n305 = local read "Blue"() -> (w40:dbl)
  n306 = local read "Blue"() -> (w46:dbl)
  n307 = local read "Green"() -> (w38:dbl)
  n308 = local read "Green"() -> (w45:dbl)
  n309 = local read "Green"() -> (w57:bool)
  n310 = local read "Red"() -> (w56:bool)
  n311 = local read "Blue"() -> (w58:bool)
  n312 = Equal?(x=w15, y=w17) -> (x = y?=w21:bool)
  n313 = Equal?(x=w17, y=w16) -> (x = y?=w22:bool)
  n314 = Greater?(x=w39, y=w47) -> (0:w44:bool)
  n315 = Equal?(x=w16, y=w15) -> (x = y?=w23:bool)
  n316 = Greater?(x=w40, y=w46) -> (0:w43:bool)
  n317 = Greater?(x=w38, y=w45) -> (0:w42:bool)
  n318 = Equal?(x=w67, y=w65) -> (x = y?=w64:bool)
  n319 = Equal?(x=w67, y=w66) -> (x = y?=w63:bool)
  n320 = Equal?(x=w66, y=w65) -> (x = y?=w62:bool)
  n321 = Or(x=w21, y=w22) -> (x .or. y?=w24:bool)
  n322 = case shown="True" "Save" {
    frame False {
    }
    frame True {
      n323 = flat-sequence {
        tunnel: [w1168] -> w629
        tunnel: w629 -> [w1258]
        frame #0 {
          w643 = ", " ("string")
          w639 = "\r\n"
          w657 = "\r\n"
          w742 = "    " ("string")
          w775 = "\r\n"
          w778 = "\r\n"
          w785 = "\r\n"
          w787 = "\r\n"
          w824 = "\r\n"
          w843 = "\r\n"
          w862 = "\r\n"
          w885 = "\r\n"
          w944 = "\r\n"
          w953 = ", " ("string")
          w957 = ", " ("string")
          w961 = ", " ("string")
          w1131 = "\r\n"
          w1137 = "\r\n"
          w1143 = "\r\n"
          w1164 = "\r\n"
          w1166 = "\r\n"
          w1190 = "\r\n"
          w1189 = "\r\n"
          # "Subtracted by one because \nchannel number in pythin starts \nfrom 0"
          n324 = Format Into String(format string="%f", "Blue") -> (resulting string=w762:string)  [unwired: 2 in, 1 out]
          n325 = Format Into String(format string="%f", "Red") -> (resulting string=w768:string)  [unwired: 2 in, 1 out]
          n326 = Format Into String(format string="%f", "Green") -> (resulting string=w765:string)  [unwired: 2 in, 1 out]
          n327 = Append True/False String(1:"Green Ch.", 2:"False" ("false string"), 3:"True" ("true string"), 4:"\"G\": " ("string (\"\")")) -> (0:w679:string)
          n328 = Append True/False String(1:"Red Ch.", 2:"False" ("false string"), 3:"True" ("true string"), 4:"\"R\": " ("string (\"\")")) -> (0:w689:string)
          n329 = Append True/False String(1:"Blue Ch.", 2:"False" ("false string"), 3:"True" ("true string"), 4:"\"B\": " ("string (\"\")")) -> (0:w675:string)
          n330 = Concatenate Strings("# Should be less than 1, close to one means close to circle shape\n# Just pass countors with higher values\nCritical_ratio_Ellipse = {\n    # In order to deactive just put zero" ("string (\"\")"), "\r\n", "    " ("string")) -> (w829:string)
          n331 = Format Into String(format string="%f", "Blue") -> (resulting string=w754:string)  [unwired: 2 in, 1 out]
          n332 = Format Into String(format string="%f", "Red") -> (resulting string=w756:string)  [unwired: 2 in, 1 out]
          n333 = Format Into String(format string="%f", "Green") -> (resulting string=w755:string)  [unwired: 2 in, 1 out]
          n334 = Concatenate Strings("    " ("string"), "\"R\":  " ("string (\"\")"), w768, "," ("string (\"\")"), "\r\n") -> (w826:string)
          n335 = Concatenate Strings("\"B\":  " ("string (\"\")"), w762, "," ("string (\"\")"), "\r\n") -> (w828:string)
          n336 = Concatenate Strings("    " ("string"), "\"G\":  " ("string (\"\")"), w765, "," ("string (\"\")"), "\r\n") -> (w827:string)
          n337 = Concatenate Strings("    " ("string"), w689, "," ("string (\"\")"), "\r\n") -> (w667:string)
          n338 = local write "Saving"(TRUE ("Saving")) -> ()
          n339 = Concatenate Strings("    " ("string"), w679, "," ("string (\"\")"), "\r\n") -> (w670:string)
          n340 = Append True/False String(1:"Green", 2:"False" ("false string"), 3:"True" ("true string"), 4:"\"G\": " ("string (\"\")")) -> (0:w919:string)
          n341 = Concatenate Strings("# It filters all contours which have perimeter to area ration greater than:\n# max-(*)std\nRemove_Ratio_Margin_ch = {" ("string (\"\")"), "\r\n", "    " ("string")) -> (w867:string)
          n342 = Concatenate Strings("\r\n", "enable_channel_for_analysis = {" ("string (\"\")"), "\r\n") -> (w668:string)
          n343 = Append True/False String(1:"Red", 2:"False" ("false string"), 3:"True" ("true string"), 4:"\"R\": " ("string (\"\")")) -> (0:w909:string)
          n344 = Concatenate Strings("    " ("string"), w675, "," ("string (\"\")"), "\r\n") -> (w669:string)
          n345 = Append True/False String(1:"Blue", 2:"False" ("false string"), 3:"True" ("true string"), 4:"\"B\": " ("string (\"\")")) -> (0:w923:string)
          n346 = Concatenate Strings("    " ("string"), "\"R\": " ("string (\"\")"), w756, "," ("string (\"\")"), "\r\n") -> (w864:string)
          n347 = Concatenate Strings("\"B\": " ("string (\"\")"), w754, "," ("string (\"\")"), "\r\n") -> (w866:string)
          n348 = Concatenate Strings("    " ("string"), "\"G\": " ("string (\"\")"), w755, "," ("string (\"\")"), "\r\n") -> (w865:string)
          n349 = call <vilib>:"Color to RGB.vi"("Color"="Blue Ch") -> ("R"=w1046:u8, "G"=w1044:u8, "B"=w1043:u8)  [unwired: 1 out]
          n350 = call <vilib>:"Color to RGB.vi"("Color"="Green Ch") -> ("R"=w1023:u8, "G"=w1025:u8, "B"=w1026:u8)  [unwired: 1 out]
          n351 = Number To Decimal String(number="Red") -> (decimal integer string=w1088:string)  [unwired: 1 in]
          n352 = Number To Decimal String(number="Blue") -> (decimal integer string=w1091:string)  [unwired: 1 in]
          n353 = call <vilib>:"Color to RGB.vi"("Color"="Red Ch") -> ("R"=w1020:u8, "G"=w1018:u8, "B"=w1017:u8)  [unwired: 1 out]
          n354 = Number To Decimal String(number="Green") -> (decimal integer string=w1090:string)  [unwired: 1 in]
          n355 = case shown="True" "Filling contours by solid color" {
            tunnel: [1 ("number") -1 ("number")] -> w1134
            frame False {
            }
            frame True {
            }
          }
          n356 = Append True/False String(1:"Activate", 2:"False" ("false string"), 3:"True" ("true string"), 4:"enable_ellipse_filter = " ("string (\"\")")) -> (0:w784:string)
          n357 = Concatenate Strings("    " ("string"), w909, "," ("string (\"\")"), "\r\n") -> (w932:string)
          n358 = Number To Decimal String(number="Red") -> (decimal integer string=w1122:string)  [unwired: 1 in]
          n359 = Number To Decimal String(number="Blue") -> (decimal integer string=w1125:string)  [unwired: 1 in]
          n360 = Number To Decimal String(number="Green") -> (decimal integer string=w1124:string)  [unwired: 1 in]
          n361 = Concatenate Strings("    " ("string"), w919, "," ("string (\"\")"), "\r\n") -> (w929:string)
          n362 = Number To Decimal String(number="Border thickness (single channel) 2") -> (decimal integer string=w945:string)  [unwired: 1 in]
          n363 = Concatenate Strings(w829, w828, w827, w826, "}" ("string"), w824, w824) -> (w822:string)
          n364 = Number To Decimal String(number="Number of bins") -> (decimal integer string=w1161:string)  [unwired: 1 in]
          n365 = Number To Decimal String(number=w1044) -> (decimal integer string=w1042:string)  [unwired: 1 in]
          n366 = Number To Decimal String(number=w1043) -> (decimal integer string=w1041:string)  [unwired: 1 in]
          n367 = Number To Decimal String(number=w1046) -> (decimal integer string=w1045:string)  [unwired: 1 in]
          n368 = Number To Decimal String(number=w1025) -> (decimal integer string=w1027:string)  [unwired: 1 in]
          n369 = Number To Decimal String(number=w1026) -> (decimal integer string=w1028:string)  [unwired: 1 in]
          n370 = call <vilib>:"Color to RGB.vi"("Color"="General border color") -> ("R"=w1158:u8, "G"=w1156:u8, "B"=w1155:u8)  [unwired: 1 out]
          n371 = Number To Decimal String(number=w1023) -> (decimal integer string=w1024:string)  [unwired: 1 in]
          n372 = Number To Decimal String(number=w1018) -> (decimal integer string=w1016:string)  [unwired: 1 in]
          n373 = Number To Decimal String(number=w1017) -> (decimal integer string=w1015:string)  [unwired: 1 in]
          n374 = Number To Decimal String(number=w1020) -> (decimal integer string=w1019:string)  [unwired: 1 in]
          n375 = Concatenate Strings(w784, w778, w778) -> (w779:string)
          n376 = Concatenate Strings("enable_adp_threshold = {" ("string (\"\")"), "\r\n") -> (w931:string)
          n377 = Concatenate Strings("    " ("string"), w923, "," ("string (\"\")"), "\r\n") -> (w930:string)
          n378 = Append True/False String(1:"Activate", 2:"False" ("false string"), 3:"True" ("true string"), 4:"# Filters\nenable_ratio_filter = " ("string (\"\")")) -> (0:w880:string)
          n379 = Concatenate Strings("# Channel color codes\nch = {" ("string (\"\")"), "\r\n") -> (w1093:string)
          n380 = Concatenate Strings(w668, w669, w670, w667, "}" ("string"), "\r\n") -> (w661:string)
          n381 = Concatenate Strings("    " ("string"), "\"R\": " ("string (\"\")"), w1088, "," ("string (\"\")"), "\r\n") -> (w1086:string)
          n382 = Concatenate Strings("    " ("string"), "\"B\": " ("string (\"\")"), w1091, "," ("string (\"\")"), "\r\n") -> (w1094:string)
          n383 = Number To Decimal String(number="Border thickness (overlay)") -> (decimal integer string=w1148:string)  [unwired: 1 in]
          n384 = Concatenate Strings("    " ("string"), "\"G\": " ("string (\"\")"), w1090, "," ("string (\"\")"), "\r\n") -> (w1095:string)
          n385 = Number To Decimal String(number="Border thickness (single channel)") -> (decimal integer string=w1144:string)  [unwired: 1 in]
          n386 = Concatenate Strings("# Contours size limits\nmin_size_limit = {" ("string (\"\")"), "\r\n") -> (w1127:string)
          n387 = Number To Decimal String(number=w1156) -> (decimal integer string=w1153:string)  [unwired: 1 in]
          n388 = Number To Decimal String(number=w1155) -> (decimal integer string=w1151:string)  [unwired: 1 in]
          n389 = Number To Decimal String(number=w1158) -> (decimal integer string=w1157:string)  [unwired: 1 in]
          n390 = Append True/False String(1:"Activate", 2:"False" ("false string"), 3:"True" ("true string"), 4:"# Generating png of interested contours\nenable_most_biggest_contours_output = " ("string (\"\")")) -> (0:w950:string)
          n391 = Concatenate Strings("    " ("string"), "\"R\": " ("string (\"\")"), w1122, "," ("string (\"\")"), "\r\n") -> (w1098:string)
          n392 = Concatenate Strings("    " ("string"), "\"B\": " ("string (\"\")"), w1125, "," ("string (\"\")"), "\r\n") -> (w1128:string)
          n393 = Concatenate Strings("    " ("string"), "\"G\": " ("string (\"\")"), w1124, "," ("string (\"\")"), "\r\n") -> (w1129:string)
          n394 = Concatenate Strings(w867, w866, w865, w864, "}" ("string"), w862, w862) -> (w860:string)
          n395 = Concatenate Strings("Channel_Border_Color = {" ("string"), "\r\n") -> (w1004:string)
          n396 = Concatenate Strings("    " ("string"), "\"B\": " ("string"), "(" ("string"), w1045, ", " ("string"), w1042, ", " ("string"), w1041, ")" ("string"), "," ("string"), "\r\n") -> (w1003:string)
          n397 = Concatenate Strings("    " ("string"), "\"G\": " ("string"), "(" ("string"), w1024, ", " ("string"), w1027, ", " ("string"), w1028, ")" ("string"), "," ("string"), "\r\n") -> (w1002:string)
          n398 = Concatenate Strings("desired_number = " ("string"), w945, w944, w944) -> (w941:string)
          n399 = Concatenate Strings(w880, "\r\n") -> (w859:string)
          n400 = Concatenate Strings("    " ("string"), "\"R\": " ("string"), "(" ("string"), w1019, ", " ("string"), w1016, ", " ("string"), w1015, ")," ("string"), "\r\n") -> (w1001:string)
          n401 = Concatenate Strings("num_bins = " ("string"), w1161, w1164, w1164) -> (w1163:string)
          n402 = Number To Decimal String(number=w1134) -> (decimal integer string=w1135:string)  [unwired: 1 in]
          n403 = Concatenate Strings(w950, "\r\n") -> (w940:string)
          n404 = Concatenate Strings("hist_subplot_indx = {" ("string (\"\")"), w1190, w742, "# You can change the order of plots" ("string"), w1190, w742) -> (w1173:string)
          n405 = Concatenate Strings("# Borders Thikness\nsingle_clr_border_thikness = " ("string"), w1148, "\r\n") -> (w1139:string)
          n406 = Concatenate Strings("full_clr_border_thikness = " ("string"), w1144, w1143, w1143) -> (w1138:string)
          n407 = Concatenate Strings("# Outline color for single channel outputs\nGenral_Borders_Color = " ("string"), "(" ("string"), w1157, ", " ("string"), w1153, ", " ("string"), w1151, ")" ("string"), w1137, w1137) -> (w1140:string)
          n408 = Concatenate Strings(w859, w860, w779) -> (w841:string)
          n409 = Concatenate Strings(w931, w930, w929, w932, "}" ("string"), "\r\n") -> (w928:string)
          n410 = Subtract(x="RED", y=1.0) -> (x-y=w630:dbl)
          n411 = Subtract(x="GREEN", y=1.0) -> (x-y=w631:dbl)
          n412 = Concatenate Strings("# Histogram setting\n# Activate histogram generator 0 or 1" ("string (\"\")"), "\r\n", "enable_hist_generator = " ("string (\"\")")) -> (w1197:string)
          n413 = Concatenate Strings(w1093, w1094, w1095, w1086, "}" ("string"), "\r\n") -> (w1052:string)
          n414 = Concatenate Strings(w1004, w1003, w1002, w1001, "}" ("string"), w785, w785) -> (w965:string)
          n415 = Subtract(x="BLUE", y=1.0) -> (x-y=w632:dbl)
          n416 = Concatenate Strings(w1127, w1128, w1129, w1098, "}" ("string"), "\r\n") -> (w1112:string)
          n417 = Concatenate Strings("# Fill inside contours\n# In order to fill put -1 otherwise 1 for outlines\nfill_black_bgd = " ("string"), w1135, "  " ("string"), "# Overlay" ("string"), w1131, w1131) -> (w1130:string)
          n418 = Number To Decimal String(number=w630) -> (decimal integer string=w642:string)  [unwired: 1 in]
          n419 = Append True/False String(1:"Activate Histogram", 2:"False" ("false string"), 3:"True" ("true string"), 4:w1197) -> (0:w1196:string)
          n420 = Number To Decimal String(number=w631) -> (decimal integer string=w644:string)  [unwired: 1 in]
          n421 = Concatenate Strings(w940, w941, w928) -> (w939:string)
          n422 = Number To Decimal String(number="Red") -> (decimal integer string=w1175:string)  [unwired: 1 in]
          n423 = Concatenate Strings("image_source_folder = \"" ("string"), "Input folder", "\"" ("string"), "\r\n") -> (w1203:string)
          n424 = Number To Decimal String(number=w632) -> (decimal integer string=w645:string)  [unwired: 1 in]
          n425 = Number To Decimal String(number="Blue") -> (decimal integer string=w1184:string)  [unwired: 1 in]
          n426 = Number To Decimal String(number="Green") -> (decimal integer string=w1183:string)  [unwired: 1 in]
          n427 = Number To Decimal String(number="To be ignored") -> (decimal integer string=w648:string)  [unwired: 1 in]
          n428 = Concatenate Strings(w1140, w1139, w1138, w1130) -> (w1110:string)
          n429 = Concatenate Strings(w1196, w1189, w1189) -> (w1193:string)
          n430 = Append True/False String(1:"Detailed output", 2:"False" ("false string"), 3:"True" ("true string"), 4:"detailed_output = " ("string (\"\")")) -> (0:w695:string)
          n431 = Append True/False String(1:"Transparent Corrector", 2:"False" ("false string"), 3:"True" ("true string"), 4:"transparent_corrector = " ("string (\"\")")) -> (0:w1221:string)
          n432 = Append True/False String(1:"Contour Detail Reporter", 2:"False" ("false string"), 3:"True" ("true string"), 4:"contours_details_reporting = " ("string (\"\")")) -> (0:w1215:string)
          n433 = Append True/False String(1:"Zero Pixel Reporter", 2:"False" ("false string"), 3:"True" ("true string"), 4:"zero_pixel_reporting = " ("string (\"\")")) -> (0:w1209:string)
          n434 = Append True/False String(1:"Green", 2:"False" ("false string"), 3:"True" ("true string"), 4:"\"G\": " ("string (\"\")")) -> (0:w803:string)
          n435 = Concatenate Strings(w1203, "\r\n") -> (w1202:string)
          n436 = Append True/False String(1:"Red", 2:"False" ("false string"), 3:"True" ("true string"), 4:"\"R\": " ("string (\"\")")) -> (0:w793:string)
          n437 = Append True/False String(1:"Blue", 2:"False" ("false string"), 3:"True" ("true string"), 4:"\"B\": " ("string (\"\")")) -> (0:w807:string)
          n438 = Concatenate Strings("    " ("string"), "\"R\": " ("string (\"\")"), w1175, "," ("string (\"\")"), "\r\n") -> (w1170:string)
          n439 = Concatenate Strings("\"B\": " ("string (\"\")"), w1184, "," ("string (\"\")"), "\r\n") -> (w1172:string)
          n440 = Concatenate Strings("    " ("string"), "\"G\": " ("string (\"\")"), w1183, "," ("string (\"\")"), "\r\n") -> (w1171:string)
          n441 = Format Into String(format string="%f", "Green") -> (resulting string=w746:string)  [unwired: 2 in, 1 out]
          n442 = Format Into String(format string="%f", "Blue") -> (resulting string=w747:string)  [unwired: 2 in, 1 out]
          n443 = Format Into String(format string="%f", "Red") -> (resulting string=w745:string)  [unwired: 2 in, 1 out]
          n444 = Number To Decimal String(number="block size") -> (decimal integer string=w655:string)  [unwired: 1 in]
          n445 = Number To Decimal String(number="Red") -> (decimal integer string=w892:string)  [unwired: 1 in]
          n446 = Number To Decimal String(number="Blue") -> (decimal integer string=w901:string)  [unwired: 1 in]
          n447 = Concatenate Strings("    " ("string"), w793, "," ("string (\"\")"), "\r\n") -> (w815:string)
          n448 = Number To Decimal String(number="Green") -> (decimal integer string=w900:string)  [unwired: 1 in]
          n449 = Concatenate Strings(w657, "# channel process" ("string"), w657, w1221, "\r\n", w1215, "\r\n", w1209, "\r\n", w695, "\r\n") -> (w700:string)
          n450 = Concatenate Strings(w639, w639, "# Channel color recepie" ("string"), w639, "ch_to_ignore = " ("string"), w648, "\r\n", "order_recepie = [" ("string"), w645, w643, w644, w643, w642, "]" ("string")) -> (w640:string)
          n451 = Number To Decimal String(number="Red") -> (decimal integer string=w1233:string)  [unwired: 1 in]
          n452 = Concatenate Strings("    " ("string"), w803, "," ("string (\"\")"), "\r\n") -> (w812:string)
          n453 = Number To Decimal String(number="Blue") -> (decimal integer string=w1230:string)  [unwired: 1 in]
          n454 = call <vilib>:"Color to RGB.vi"("Color"="Blue Ch") -> ("R"=w967:u8, "G"=w969:u8, "B"=w970:u8)  [unwired: 1 out]
          n455 = Number To Decimal String(number="Green") -> (decimal integer string=w1231:string)  [unwired: 1 in]
          n456 = call <vilib>:"Color to RGB.vi"("Color"="Green Ch") -> ("R"=w985:u8, "G"=w983:u8, "B"=w982:u8)  [unwired: 1 out]
          n457 = Number To Decimal String(number="Red") -> (decimal integer string=w1058:string)  [unwired: 1 in]
          n458 = Number To Decimal String(number="Blue") -> (decimal integer string=w1056:string)  [unwired: 1 in]
          n459 = call <vilib>:"Color to RGB.vi"("Color"="Red Ch") -> ("R"=w988:u8, "G"=w990:u8, "B"=w991:u8)  [unwired: 1 out]
          n460 = Number To Decimal String(number="Green") -> (decimal integer string=w1057:string)  [unwired: 1 in]
          n461 = Concatenate Strings("# Contour remover by number filter\nenable_selection_filter = {" ("string (\"\")"), "\r\n") -> (w814:string)
          n462 = Concatenate Strings("# Should be less than 1, close to one means circle is filled more\n# Just pass countors with higher values\nCritical_ratio_Circle = {\n    # In order to deactive just put zero" ("string (\"\")"), "\r\n", "    " ("string")) -> (w848:string)
          n463 = Concatenate Strings("    " ("string"), w807, "," ("string (\"\")"), "\r\n") -> (w813:string)
          n464 = Concatenate Strings("\r\n", "# adaptive threshold\nblock_size = " ("string (\"\")"), w655) -> (w653:string)
          n465 = Concatenate Strings("Adp_Threshold_vals = {" ("string (\"\")"), "\r\n", "    " ("string")) -> (w890:string)
          n466 = Concatenate Strings(w1173, w1172, w1171, w1170, "}" ("string"), w1166, w1166, w1163) -> (w1167:string)
          n467 = Concatenate Strings("    " ("string"), "\"R\": " ("string (\"\")"), w745, "," ("string (\"\")"), "\r\n") -> (w845:string)
          n468 = Concatenate Strings("\"B\": " ("string (\"\")"), w747, "," ("string (\"\")"), "\r\n") -> (w847:string)
          n469 = Concatenate Strings("    " ("string"), "\"G\": " ("string (\"\")"), w746, "," ("string (\"\")"), "\r\n") -> (w846:string)
          n470 = Number To Decimal String(number=w969) -> (decimal integer string=w971:string)  [unwired: 1 in]
          n471 = Number To Decimal String(number=w970) -> (decimal integer string=w962:string)  [unwired: 1 in]
          n472 = Number To Decimal String(number=w967) -> (decimal integer string=w968:string)  [unwired: 1 in]
          n473 = Number To Decimal String(number=w983) -> (decimal integer string=w981:string)  [unwired: 1 in]
          n474 = Number To Decimal String(number=w982) -> (decimal integer string=w980:string)  [unwired: 1 in]
          n475 = Concatenate Strings("    " ("string"), "\"R\": " ("string (\"\")"), w892, "," ("string (\"\")"), "\r\n") -> (w887:string)
          n476 = Number To Decimal String(number=w985) -> (decimal integer string=w984:string)  [unwired: 1 in]
          n477 = Concatenate Strings("\"B\": " ("string (\"\")"), w901, "," ("string (\"\")"), "\r\n") -> (w889:string)
          n478 = Number To Decimal String(number=w990) -> (decimal integer string=w992:string)  [unwired: 1 in]
          n479 = Number To Decimal String(number=w991) -> (decimal integer string=w993:string)  [unwired: 1 in]
          n480 = Number To Decimal String(number=w988) -> (decimal integer string=w989:string)  [unwired: 1 in]
          n481 = Concatenate Strings("    " ("string"), "\"G\": " ("string (\"\")"), w900, "," ("string (\"\")"), "\r\n") -> (w888:string)
          n482 = Concatenate Strings("    " ("string"), "\"R\": " ("string (\"\")"), w1233, "," ("string (\"\")"), "\r\n") -> (w1101:string)
          n483 = Concatenate Strings("max_size_limit = {" ("string (\"\")"), "\r\n") -> (w1228:string)
          n484 = Concatenate Strings("# These are static threshold and when adaptive filter is\n# off these thresholds apply automatically\nThreshold_vals = {" ("string (\"\")"), "\r\n") -> (w1055:string)
          n485 = Concatenate Strings("    " ("string"), "\"B\": " ("string (\"\")"), w1230, "," ("string (\"\")"), "\r\n") -> (w1227:string)
          n486 = Concatenate Strings("    " ("string"), "\"G\": " ("string (\"\")"), w1231, "," ("string (\"\")"), "\r\n") -> (w1226:string)
          n487 = Format Into String(format string="%.;%f", "Overlay Transparency") -> (resulting string=w771:string)  [unwired: 2 in, 1 out]
          n488 = Concatenate Strings("    " ("string"), "\"R\": " ("string (\"\")"), w1058, "," ("string (\"\")"), "\r\n") -> (w1059:string)
          n489 = Concatenate Strings("    " ("string"), "\"B\": " ("string (\"\")"), w1056, "," ("string (\"\")"), "\r\n") -> (w1054:string)
          n490 = Concatenate Strings("    " ("string"), "\"G\": " ("string (\"\")"), w1057, "," ("string (\"\")"), "\r\n") -> (w1053:string)
          n491 = Concatenate Strings("Channel_Border_Color_tr = {" ("string"), "\r\n") -> (w997:string)
          n492 = Concatenate Strings("    " ("string"), "\"B\": " ("string"), "(" ("string"), w968, ", " ("string"), w971, w961, w962, w961, "0" ("string"), ")," ("string"), "\r\n") -> (w998:string)
          n493 = Concatenate Strings("    " ("string"), "\"G\": " ("string"), "(" ("string"), w984, ", " ("string"), w981, w957, w980, w957, "0" ("string"), ")," ("string"), "\r\n") -> (w999:string)
          n494 = Concatenate Strings("    " ("string"), "\"R\": " ("string"), "(" ("string"), w989, ", " ("string"), w992, w953, w993, w953, "0" ("string"), ")," ("string"), "\r\n") -> (w1000:string)
          n495 = Concatenate Strings(w814, w813, w812, w815, "}" ("string"), "\r\n") -> (w790:string)
          n496 = Concatenate Strings(w822, w790) -> (w820:string)
          n497 = Concatenate Strings("overlay_transparency = " ("string"), w771, "  # Is used for combined image" ("string"), w775, w775) -> (w776:string)
          n498 = Concatenate Strings(w848, w847, w846, w845, "}" ("string"), w843, w843) -> (w821:string)
          n499 = call "Time Delay"("Delay Time (s)"=0.05) -> ()  [unwired: 10 in, 1 out]
          n500 = Concatenate Strings(w890, w889, w888, w887, "}" ("string"), w885, w885) -> (w883:string)
          n501 = Concatenate Strings(w1228, w1227, w1226, w1101, "}" ("string"), "\r\n") -> (w1111:string)
          n502 = Concatenate Strings(w700, w661, w653, w640) -> (w701:string)
          n503 = Concatenate Strings(w1055, w1054, w1053, w1059, "}" ("string"), "\r\n") -> (w1051:string)
          n504 = Concatenate Strings(w997, w998, w999, w1000, "}" ("string"), w787, w787, w776) -> (w964:string)
          n505 = Concatenate Strings(w965, w964, w939, w883) -> (w963:string)
          n506 = Concatenate Strings(w841, w821, w820) -> (w840:string)
          n507 = Concatenate Strings(w1112, w1111, w1052, w1051, w963, w840) -> (w1108:string)
          n508 = Concatenate Strings(w1110, w1108) -> (w1109:string)
          n509 = Concatenate Strings(w1202, w1193, w1167, w1109, w701) -> (w1168:string)
        }
        frame #1 {
          n510 = Current VI's Path() -> (path=w1246:path)
          n511 = Strip Path(path=w1246) -> (stripped path=w1248:path)  [unwired: 1 out]
          n512 = Build Path(base path=w1248, name or relative path=path "setting_batch.py") -> (appended path=w1245:path)
          n513 = local read "messages"() -> (w1250:string)
          n514 = Open/Create/Replace File(file path (use dialog)=w1245, operation (0:open)=T4."replace or create") -> (refnum out=w1261:refnum<file>)  [unwired: 4 in, 2 out]
          n515 = local write "Scroll to last"(TRUE ("Scroll to last")) -> ()
          n516 = Get Date/Time In Seconds() -> (seconds since 1Jan1904=w1255:timestamp)
          n517 = Write to Text File(file (use dialog)=w1261, text=w1258) -> (refnum out=w1260:refnum<file>)  [unwired: 2 in, 2 out]
          n518 = local write "Saving"(FALSE ("Saving")) -> ()
          n519 = Format Date/Time String(time format string (%c)="(%m/%d/%Y - %H:%M:%S) ", seconds (now)=w1255) -> (date/time string=w1254:string)  [unwired: 1 in]
          n520 = Close File(refnum=w1260) -> ()  [unwired: 1 in, 2 out]
          n521 = Concatenate Strings(w1250, "\r\n", w1254, "Setting sucessfully saved.") -> (w1251:string)
          n522 = local write "messages"(w1251) -> ()
        }
      }
    }
  }
  n523 = Or(x=w44, y=w43) -> (x .or. y?=w41:bool)
  n524 = Or(x=w64, y=w63) -> (x .or. y?=w61:bool)
  n525 = Or(x=w58, y=w57) -> (x .or. y?=w55:bool)
  n526 = case shown="True" "Run" {
    frame False {
    }
    frame True {
      n527 = stacked-sequence {
        frame #0 {
          n528 = local read "messages"() -> (w1265:string)
          n529 = local write "Scroll to last"(TRUE ("Scroll to last")) -> ()
          n530 = Concatenate Strings(w1265, "\r\n", " Python is running, please wait  ..." ("string")) -> (w1266:string)
          n531 = local write "messages"(w1266) -> ()
        }
        frame #1 {
          n532 = Current VI's Path() -> (path=w1268:path)
          n533 = Strip Path(path=w1268) -> (stripped path=w1270:path)  [unwired: 1 out]
          n534 = Build Path(base path=w1270, name or relative path=path "filter_batch_labview.py") -> (appended path=w1267:path)
          n535 = Open Python Session(python version="Python version") -> (session out=w1273:refnum<k35>, error out=w1274:errorcluster)  [unwired: 2 in]
          n536 = node(w1273, w1267, "run" ("function name"), w1274) -> (w1275:refnum<k35>, w1276:errorcluster)  [unwired: 2 in, 2 out]
          n537 = Close Python Session(session in=w1275, error in=w1276) -> ()  [unwired: 1 out]
          n538 = local write "Processing"(TRUE ("Boolean")) -> ()
        }
        frame #2 {
          n539 = local write "Scroll to last"(TRUE ("Scroll to last")) -> ()
          n540 = local write "Processing"(FALSE ("Boolean")) -> ()
          n541 = local read "messages"() -> (w1281:string)
          n542 = Concatenate Strings(w1281, "\r\n", " Process is done sucessfully." ("string")) -> (w1282:string)
          n543 = local write "messages"(w1282) -> ()
        }
      }
    }
  }
  n544 = Or(x=w24, y=w23) -> (x .or. y?=w9:bool)
  n545 = Or(x=w55, y=w56) -> (x .or. y?=w52:bool)
  n546 = property on="Warning" class="Bool (strict)"("Blinking"=w52) -> ()  [unwired: 2 in, 2 out]
  n547 = Or(x=w9, y=w10) -> (x .or. y?=w8:bool)
  n548 = Or(x=w41, y=w42) -> (x .or. y?=w48:bool)
  n549 = Or(x=w61, y=w62) -> (x .or. y?=w30:bool)
  n550 = case shown="True" "Remove Button" {
    frame False {
    }
    frame True {
      n551 = local write "messages"("" ("Warning and error window 2")) -> ()
    }
  }
  n552 = case shown="True" w8 {
    tunnel: ["" ("Warning and error window") w1287] -> w18
    tunnel: [FALSE ("Setting error") TRUE ("Setting error")] -> w20
    frame False {
    }
    frame True {
      n553 = Concatenate Strings("Error: You cannot use the same channel for different colors" ("Warning and error window"), "\r\n") -> (w1287:string)
    }
  }
  n554 = case shown="True" w48 {
    tunnel: ["" ("Warning and error window") w1293] -> w31
    tunnel: [FALSE ("Setting error") TRUE ("Setting error")] -> w36
    frame False {
    }
    frame True {
      n555 = Concatenate Strings("Error: Minimum size limit is greater that the maximum limit!" ("Warning and error window"), "\r\n") -> (w1293:string)
    }
  }
  n556 = case shown="True" w30 {
    tunnel: ["" ("Warning and error window") w1299] -> w54
    tunnel: [FALSE ("Setting error") TRUE ("Setting error")] -> w37
    frame False {
    }
    frame True {
      n557 = Concatenate Strings("Error: Order of plot for each color should be specific!" ("Warning and error window"), "\r\n") -> (w1299:string)
    }
  }
  n558 = case shown="False" w52 {
    tunnel: [FALSE ("Setting error") TRUE ("Setting error")] -> w51
    tunnel: ["" ("Warning and error window") w1305] -> w32
    frame False {
    }
    frame True {
      n559 = Concatenate Strings("Warning: When you enable selection filter please run the filter.py directly in terminal and prepare your text file in root as instruction said. " ("Warning and error window"), "\r\n") -> (w1305:string)
    }
  }
  n560 = Or(x=w37, y=w36) -> (x .or. y?=w19:bool)
  n561 = Or(x=w19, y=w20) -> (x .or. y?=w7:bool)
  n562 = Concatenate Strings(w54, w31, w18) -> (w35:string)
  n563 = Concatenate Strings(w32) -> (w34:string)
  n564 = Concatenate Strings(w35, w34) -> (w33:string)
  n565 = case shown="True" "Scroll to last" {
    frame False {
    }
    frame True {
      n566 = local read "messages"() -> (w1312:string)
      "messages" <- w1312
      n567 = String Length(string=w1312) -> (length=w1309:i32)
      n568 = for {
        N: w1309 -> [_]
        tunnel: w1312 -> [w1323]
        shift-right: [w1321] -> w1311
        shift-left: "Initial Scroll Position" -> [w1313]
        i -> [w1324]
        n569 = String Subset(string=w1323, offset (0)=w1324, length (rest)=1 ("length (rest)")) -> (substring=w1319:string)
        n570 = Match Pattern(string=w1319, regular expression="\n") -> (offset past match=w1318:i32)  [unwired: 1 in, 3 out]
        n571 = Match Pattern(string=w1319, regular expression="\r") -> (offset past match=w1322:i32)  [unwired: 1 in, 3 out]
        n572 = Less Than 0?(x=w1322) -> (x < 0?=w1316:bool)
        n573 = Less Than 0?(x=w1318) -> (x < 0?=w1315:bool)
        n574 = Not Exclusive Or(1:w1315, 2:w1316) -> (0:w1314:bool)
        n575 = case shown="False" w1314 {
          tunnel: [w1326 w1328] -> w1321
          tunnel: w1313 -> [w1327 w1328]
          frame False {
            n576 = Increment(x=w1327) -> (x+1=w1326:u32)
            n577 = local write "Final Scroll Position"(w1326) -> ()
          }
          frame True {
          }
        }
      }
      "Final Scroll Position" <- w1311
      n578 = property on="messages" class="Str"("Text.Scroll Position"=w1311) -> ()  [unwired: 2 in, 2 out]
    }
  }
  n579 = local write "Error"(w7) -> ()
  n580 = property on="Error" class="Bool (strict)"("Blinking"=w7) -> ()  [unwired: 2 in, 2 out]
  n581 = local write "Warning"(w51) -> ()
  n582 = local write "Warning and error window"(w33) -> ()
  "Processing" <- FALSE ("Boolean")
  "Saving" <- FALSE ("Saving")
  "Error" <- FALSE ("Setting error")
  "Warning" <- FALSE ("Warning")
